vi "torque test 2.vi"() -> ()   [LabVIEW 2025]
uses:
  Libraries/Torque Transducer/Torque Transducer.lvlib
panel:
  in  "Slide":dbl(slide)=85.43417366946778 scale=0.0..100.0
  out "Waveform Chart":dbl(graph)
  out "error out":errorcluster
  in  "stop":bool
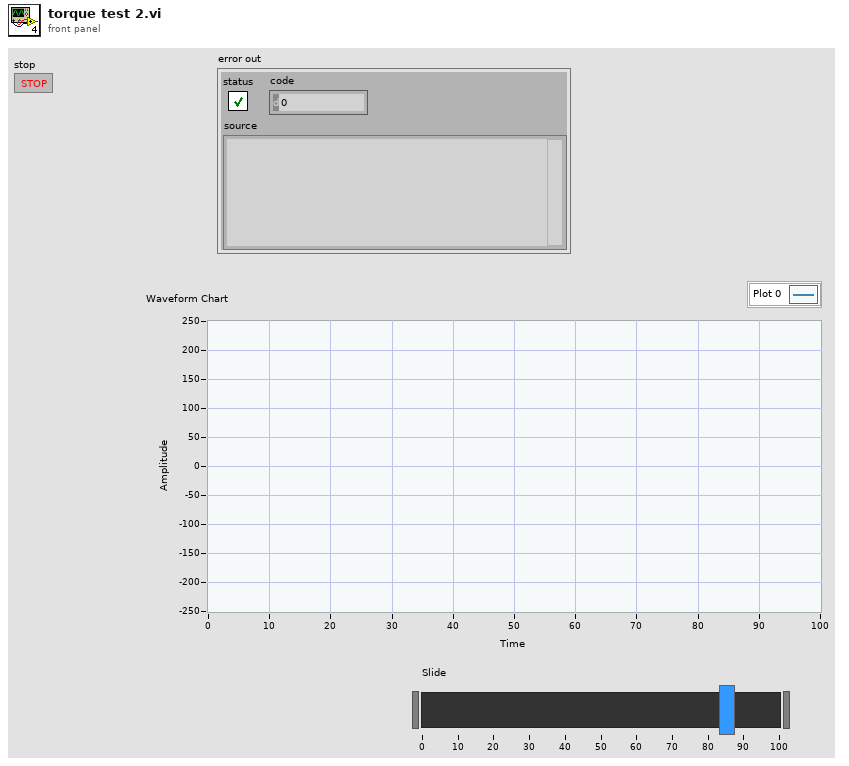
[diagram p1: front panel]
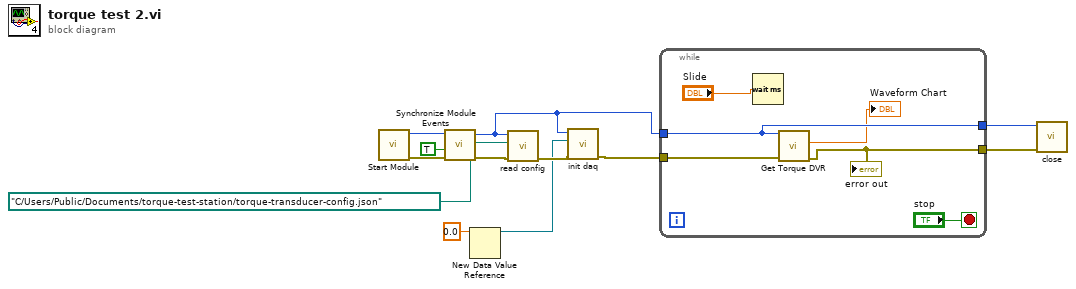
[diagram p0: block diagram]
diagram:
  n1 = call "Start Module.vi"() -> ("error out"=w11:errorcluster, "Module ID"=w12:i32)  [unwired: 7 in, 3 out]
  n2 = call "Synchronize Module Events.vi"("error in"=w11, "Wait for Event Sync?"=TRUE, "Module ID in"=w12) -> ("error out"=w7:errorcluster, "Module ID out"=w2:i32)  [unwired: 7 in]
  n3 = New Data Value Reference(data value=0.0) -> (data value reference=w3:refnum<data-value>)  [unwired: 1 in, 1 out]
  n4 = call "read config.vi"("error in"=w7, "config file path"=path "C:/Users/Public/Documents/torque-test-station/torque-transducer-config.json", "Module ID"=w2) -> ("error out"=w5:errorcluster)  [unwired: 7 in, 1 out]
  n5 = call "init daq.vi"("error in"=w5, "Torque Value"=w3, "Module ID"=w2) -> ("error out"=w1:errorcluster)  [unwired: 7 in, 1 out]
  n6 = while {
    tunnel: w2 -> [w17]
    tunnel: w1 -> [w18]
    tunnel: [w17] -> w9
    tunnel: [w16] -> w8
    stop <- "stop" stop-if-true
    n7 = Wait (ms)(milliseconds to wait="Slide") -> ()  [unwired: 1 out]
    n8 = call "Get Torque DVR.vi"("error in"=w18, "Module ID"=w17) -> ("error out"=w16:errorcluster, "Numeric"=→"Waveform Chart":dbl)  [unwired: 6 in, 2 out]
    "error out" <- w16
  }
  n9 = call "close.vi"("error in"=w8, "Module ID"=w9) -> ()  [unwired: 8 in, 2 out]
